vi "RUN_control.vi"(4 "error in":errorcluster, 5 "RUN Ref.":refnum<vi>, 6 "Blinking(:T)":bool=TRUE, 7 "Value (:T)":bool=TRUE) -> (0 "error out":errorcluster, 2 "Old Blinking":bool=TRUE, 3 "Old Value":bool=TRUE)   [LabVIEW 2017]
panel:
  in  "Add/Sub":cluster{"Left":i32, "Top":i32}
  out "RUN Pos.":cluster{"Left":i32, "Top":i32}
  in  "New RUN Pos.":cluster{"Left":i32, "Top":i32}
  out "error out 2":errorcluster
  out "RUN":bool
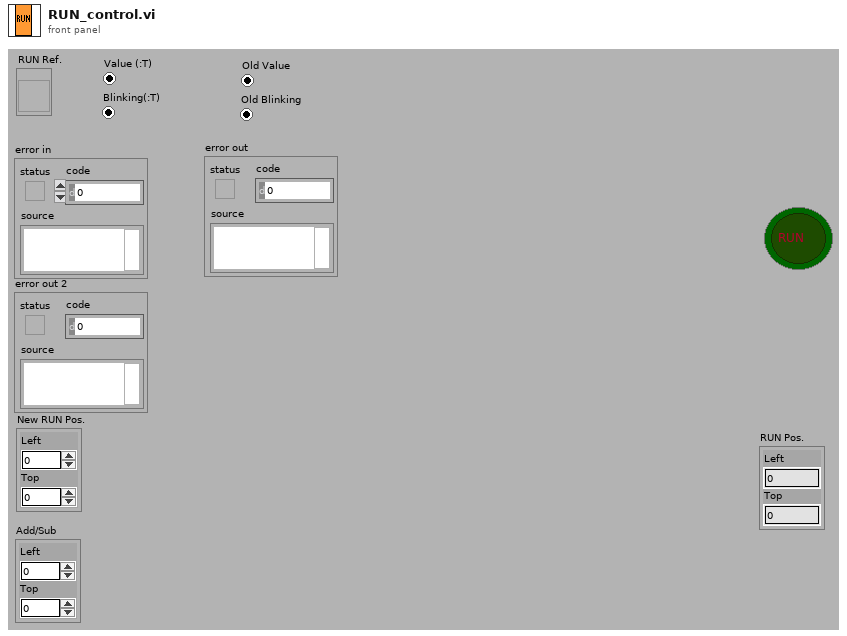
[diagram p1: front panel]
types:
  T1 = typedef "LVPositionTypeDef.ctl" = cluster{"Left":i32, "Top":i32}
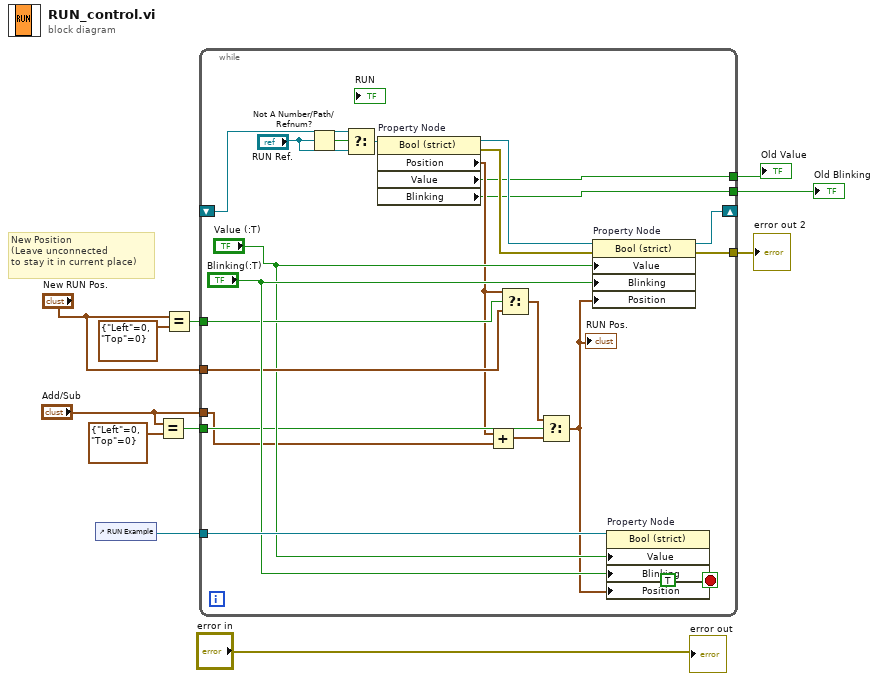
[diagram p0: block diagram]
diagram:
  # "New Position\n(Leave unconnected\nto stay it in current place)"
  n1 = control-ref of="RUN Example"() -> (w10:refnum<vi>)
  n2 = Equal?(x="Add/Sub", y=cluster{"Left":i32, "Top":i32} {"Left"=0, "Top"=0} ("Position")) -> (x = y?=w3:bool)
  n3 = Equal?(x="New RUN Pos.", y=cluster{"Left":i32, "Top":i32} {"Left"=0, "Top"=0} ("Position")) -> (x = y?=w7:bool)
  n4 = while {
    shift-right: [w26] -> _
    shift-left: _ -> [w32]
    tunnel: w10 -> [w30]
    tunnel: [w24] -> w9
    tunnel: w7 -> [w23]
    tunnel: "New RUN Pos." -> [w22]
    tunnel: "Add/Sub" -> [w15]
    tunnel: w3 -> [w18]
    tunnel: [w13] -> w2
    tunnel: [w12] -> w1
    stop <- TRUE stop-if-true
    n5 = Not A Number/Path/Refnum?(number/path/refnum="RUN Ref.") -> (NaN/Path/Refnum?=w33:bool)
    n6 = Select(t=w32, s=w33, f="RUN Ref.") -> (s? t:f=w28:refnum<vi>)
    n7 = property on="Property Node" class="Bool (strict)"(reference=w28) -> (reference out=w27:refnum<vi>, error out=w25:errorcluster, "Position"=w16:T1, "Value"=w13:bool, "Blinking"=w12:bool)  [unwired: 1 in]
    n8 = Add(x=w16, y=w15) -> (x+y=w17:T1)
    n9 = Select(t=w16, s=w23, f=w22) -> (s? t:f=w19:T1)
    n10 = Select(t=w19, s=w18, f=w17) -> (s? t:f=w14:T1)
    "RUN Pos." <- w14
    n11 = property on="Property Node" class="Bool (strict)"(reference=w27, error in=w25, "Value"="Value (:T)", "Blinking"="Blinking(:T)", "Position"=w14) -> (reference out=w26:refnum<vi>, error out=w24:errorcluster)
    n12 = property on="Property Node" class="Bool (strict)"(reference=w30, "Value"="Value (:T)", "Blinking"="Blinking(:T)", "Position"=w14) -> ()  [unwired: 1 in, 2 out]
  }
  "error out 2" <- w9
  "Old Value" <- w2
  "Old Blinking" <- w1
  "error out" <- "error in"
